vi "R Scale Range Increment Read.vi"(4 "error in (no error)":errorcluster, 6 "Container State":T3, 7 "Display State In":T1) -> (0 "error out":errorcluster, 2 "Value":dbl, 3 "Display State Out":T1)   [LabVIEW 2017, in "2D Compass.xctl"]
uses:
  <vilib>/Math Plots/2D Math Plots/2D Compass/2D Compass XCtrl/2D Compass.xctl
  <vilib>/_xctls/Container State.ctl
  <vilib>/Math Plots/2D Math Plots/2D Compass/2D Compass XCtrl/State.ctl
  <vilib>/Math Plots/2D Math Plots/2D Compass/2D Compass/2D Compass.lvclass
  <vilib>/Math Plots/2D Math Plots/2D Plot/Action String/2DMathPlot Ctrl Act Queue.ctl
  <vilib>/Math Plots/2D Math Plots/2D Plot/Action String/2DMathPlot Ctrl Act Cluster.ctl
  <vilib>/Math Plots/2D Math Plots/2D Plot/Action String/2DMathPlot State Class.ctl
  <vilib>/Math Plots/2D Math Plots/2D Plot/2D Plot/2D Plot.lvclass
  <vilib>/_xctls/XControlSupport.lvlib
panel:
  # "Replace the Value Indicator below with an Indicator of desired type.\nDo not remove this Indicator or the others from the connector pane. \nDo not change the connector pane pattern.\nThe Value Indicator should always be the second terminal from top on the output side in the connector pane."
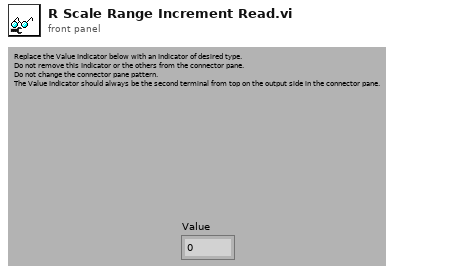
[diagram p1: front panel]
types:
  T1 = typedef "2D Compass.xctl/State.ctl" = cluster{"2D Compass.lvclass":refnum<class "2D Compass.lvclass">, "Control Ref Queue":T2, "Main Frame Color":u32, "Plot Legend Color":u32}
  T2 = typedef "2DMathPlot Ctrl Act Queue.ctl" = refnum<queue>
  T3 = typedef "XControlSupport.lvlib/Container State.ctl" = cluster{"Indicator?":bool, "Run Mode?":bool, " Refnum":refnum<vi>}
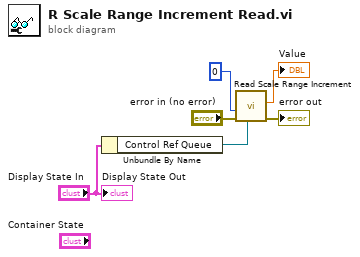
[diagram p0: block diagram]
diagram:
  n1 = Unbundle By Name("Display State In") -> ("Control Ref Queue"=w1:T2)
  n2 = call <vilib>:"Read Scale Range Increment.vi"("Control Ref Queue"=w1, "error in (no error)"="error in (no error)", "Index"=0) -> ("error out"=→"error out":errorcluster, "Increment"=→"Value":dbl)  [unwired: 1 in, 6 out]
  "Display State Out" <- "Display State In"
